vi "Serial_Write_and_ReadBack.vi"(6 "Error IN":errorcluster, 8 "Command":string, 9 "VISA Resource IN":refnum<visa-resource-name>) -> (0 "Error OUT":errorcluster, 2 "Response":string, 3 "Visa Resource OUT":refnum<visa-resource-name>)   [LabVIEW 2013]
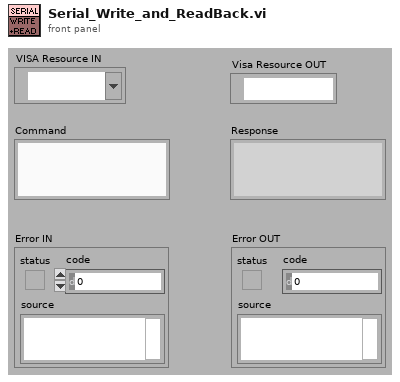
[diagram p1: front panel]
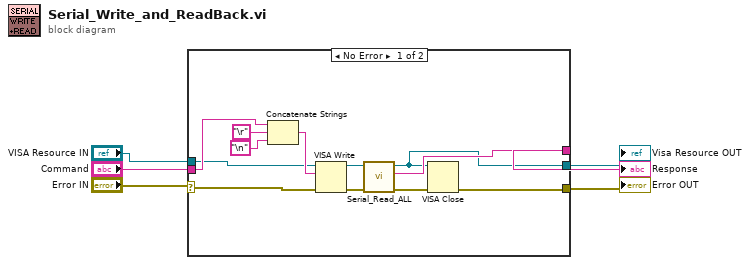
[diagram p0: block diagram]
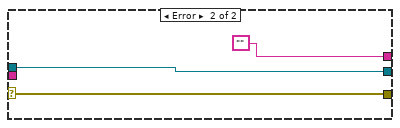
[diagram p2: hidden frame]
diagram:
  n1 = case shown="No Error" "Error IN" {
    selector: "Error IN" -> [w7 w21]
    tunnel: [w18 w21] -> w6
    tunnel: [w17 ""] -> w5
    tunnel: "Command" -> [w13 _]
    tunnel: "VISA Resource IN" -> [w8 w20]
    tunnel: [w9 w20] -> w2
    frame No Error {
      n2 = Concatenate Strings(w13, "\r", "\n") -> (w16:string)
      n3 = VISA Write(VISA resource name=w8, write buffer=w16, error in (no error)=w7) -> (VISA resource name out=w11:refnum<visa-resource-name>, error out=w12:errorcluster)  [unwired: 1 out]
      n4 = call "Serial_Read_ALL.vi"("Error IN"=w12, "Visa Resource IN"=w11) -> ("Error OUT"=w10:errorcluster, "String"=w17:string, "Visa Resource OUT"=w9:refnum<visa-resource-name>)  [unwired: 5 out]
      n5 = VISA Close(VISA resource name=w9, error in (no error)=w10) -> (error out=w18:errorcluster)
    }
    frame Error {
    }
  }
  "Error OUT" <- w6
  "Response" <- w5
  "Visa Resource OUT" <- w2
